vi "Set Active User Machine Input.vi"() -> (3 "Machine Out":string)   [LabVIEW 2016]
panel:
  in  "OK Button":bool
  in  "Which machine are you using?":string(combo)
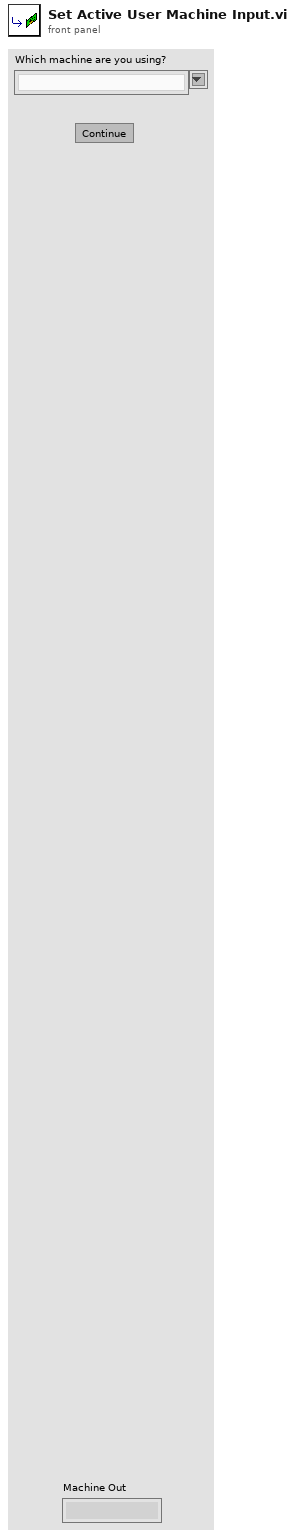
[diagram p1: front panel]
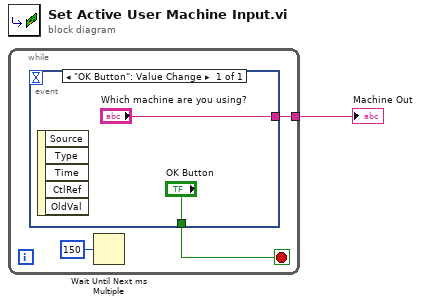
[diagram p0: block diagram]
diagram:
  n1 = while {
    tunnel: [w4] -> w1
    stop <- w3 stop-if-true
    n2 = event shown="[0] \"OK Button\": Value Change" {
      selector: _ -> [_]
      dyn-events: _ -> [_]
      timeout: _ -> [_]
      tunnel: ["Which machine are you using?"] -> w4
      tunnel: ["OK Button"] -> w3
      event "OK Button": Value Change {
        n3 = event-data() -> ()  [unwired: 1 in, 5 out]
      }
    }
    n4 = Wait Until Next ms Multiple(millisecond multiple=u32 150) -> ()  [unwired: 1 out]
  }
  "Machine Out" <- w1
